vi "Constructor.vi"(8 "error in (no error)":errorcluster, 11 "NMR in":refnum<class "NMR.lvclass">) -> (0 "error out":errorcluster, 3 "NMR out":refnum<class "NMR.lvclass">)   [LabVIEW 2011, in "NMR.lvclass"]
uses:
  NMR.lvclass
  Communication Channel.ctl
  NMR.lvclass/NMR.ctl
  <vilib>/Instr/_visa.llb/VISA Configure Serial Port (Serial Instr).vi
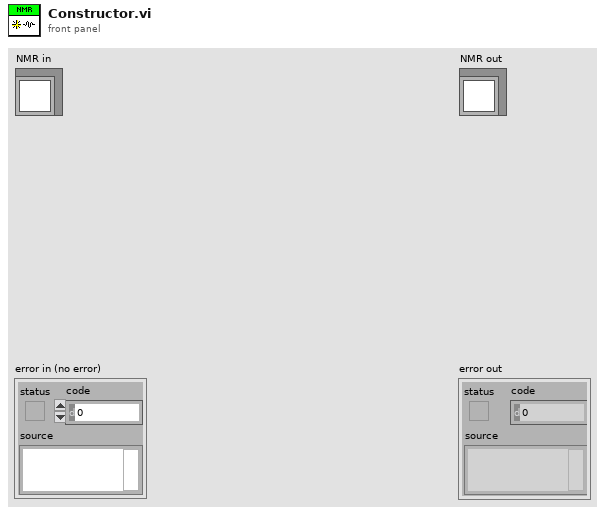
[diagram p1: front panel]
types:
  T1 = typedef "NMR.lvclass/Communication Channel.ctl" = enum16{"VISA", "DLL"}
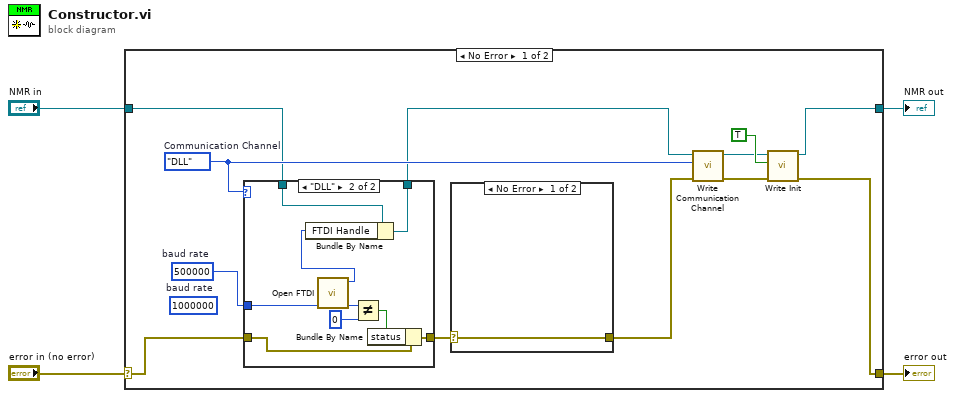
[diagram p0: block diagram]
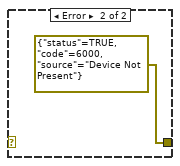
[diagram p2: hidden frame]
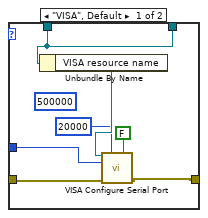
[diagram p3: hidden frame]
diagram:
  n1 = case shown="No Error" "error in (no error)" {
    selector: "error in (no error)" -> [w13 w36]
    tunnel: [w16 w36] -> w3
    tunnel: [w14 w35] -> w1
    tunnel: "NMR in" -> [w7 w35]
    frame No Error {
      w5 = u32 500000  # baud rate
      (unwired) u32 1000000  # baud rate
      w12 = Communication_Channel."DLL"  # Communication Channel
      n2 = case shown="\"DLL\"" w12 {
        tunnel: w13 -> [w25 w29]
        tunnel: [w24 w31] -> w9
        tunnel: w7 -> [w19 w33]
        tunnel: w5 -> [w20 w34]
        tunnel: [w19 w26] -> w6
        frame "VISA", Default {
          (unwired) u32 500000 ("baud rate (9600)")
          n3 = Unbundle By Name(w19) -> ("VISA resource name"=w23:refnum<visa-resource-name>)
          n4 = call-poly "VISA Configure Serial Port"("VISA resource name"=w23, "timeout (10sec)"=u32 20000, "Enable Termination\nChar (T)"=FALSE ("Enable Termination\nChar (T)"), "baud rate (9600)"=w20, "error in (no error)"=w25) -> ("error out"=w24:errorcluster)  [unwired: 9 in, 1 out]
        }
        frame "DLL" {
          n5 = call "Open FTDI.vi"("Baud Rate"=w34) -> ("FT_Status"=w27:u32, "FTDI Handle"=w32:u32)  [unwired: 9 in]
          n6 = Bundle By Name(cluster=w33, "FTDI Handle"=w32) -> (w26:refnum<class "NMR.lvclass">)
          n7 = Not Equal?(x=w27, y=u32 0) -> (x != y?=w30:bool)
          n8 = Bundle By Name(cluster=w29, "status"=w30) -> (w31:errorcluster)
        }
      }
      n9 = case shown="No Error" w9 {
        selector: w9 -> [w17 _]
        tunnel: [w17 errorcluster {"status"=TRUE, "code"=6000, "source"="Device Not Present"} ("error IO")] -> w8
        frame No Error {
        }
        frame Error {
        }
      }
      n10 = call-dynamic "Write Communication Channel.vi"("error in (no error)"=w8, "Communication Channel"=w12, "NMR in"=w6) -> ("error out"=w10:errorcluster, "NMR out"=w11:refnum<class "NMR.lvclass">)  [unwired: 7 in]
      n11 = call-dynamic "Write Init.vi"("error in (no error)"=w10, "Init"=TRUE, "NMR in"=w11) -> ("error out"=w16:errorcluster, "NMR out"=w14:refnum<class "NMR.lvclass">)  [unwired: 7 in]
    }
    frame Error {
    }
  }
  "error out" <- w3
  "NMR out" <- w1
